vi "mtg reader - recolor file list.vi"(6 "max index":i32, 8 "rowsize":i32=6, 9 "Row":i32, 10 "Column":i32, 11 "table ref":refnum<vi>) -> (2 "slider pos":i32, 3 "table ref out":refnum<vi>)   [LabVIEW 2025]
uses:
  <vilib>/Utility/miscctls.llb/LVRowAndColumnTypeDef.ctl
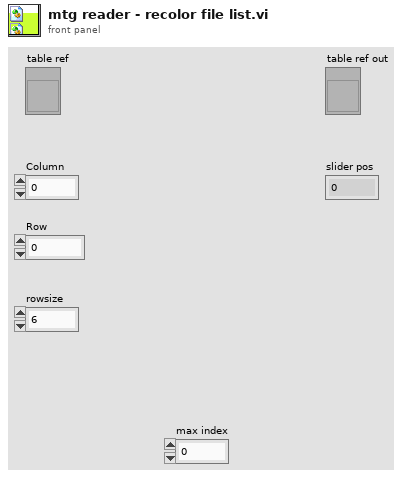
[diagram p1: front panel]
types:
  T1 = typedef "LVRowAndColumnTypeDef.ctl" = cluster{"Row":i32, "Column":i32}
  T2 = typedef "LVRowAndColumnUnsignedTypeDef.ctl" = cluster{"Row":u32, "Column":u32}
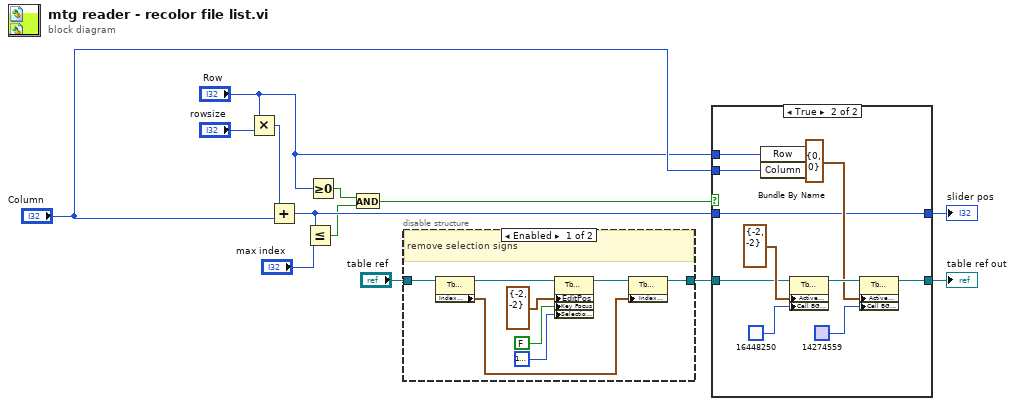
[diagram p0: block diagram]
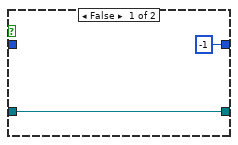
[diagram p3: hidden frame]
diagram:
  n1 = Multiply(x="Row", y="rowsize") -> (x*y=w12:i32)
  n2 = Add(x=w12, y="Column") -> (x+y=w9:i32)
  n3 = Less Or Equal?(x=w9, y="max index") -> (x <= y?=w5:bool)
  n4 = Greater Or Equal To 0?(x="Row") -> (x >= 0?=w4:bool)
  n5 = And(x=w4, y=w5) -> (x .and. y?=w6:bool)
  n6 = disable-structure shown="Enabled" {
    disable-tunnel: "table ref" -> [w18 w22]
    disable-tunnel: [w15 w22] -> w1
    frame Enabled {
      # "remove selection signs"
      n7 = property class="Tbl (strict)"(reference=w18) -> (reference out=w17:refnum<vi>, "Index Values"=w14:T2)  [unwired: 1 in, 1 out]
      n8 = property class="Tbl (strict)"(reference=w17, "EditPos"=T1 {"Row"=-2, "Column"=-2} ("Edit Position"), "Key Focus"=FALSE, "Selection Color"=u32 16777216) -> (reference out=w16:refnum<vi>)  [unwired: 1 in, 1 out]
      n9 = property class="Tbl (strict)"(reference=w16, "Index Values"=w14) -> (reference out=w15:refnum<vi>)  [unwired: 1 in, 1 out]
    }
    frame Disabled {
    }
  }
  n10 = case shown="True" w6 {
    tunnel: w1 -> [w24 w25]
    tunnel: [w24 w29] -> w3
    tunnel: "Row" -> [_ w28]
    tunnel: "Column" -> [_ w27]
    tunnel: w9 -> [_ w26]
    tunnel: [-1 w26] -> w8
    frame False {
    }
    frame True {
      n11 = Bundle By Name(cluster=T1 {"Row"=0, "Column"=0} ("Active Cell:Active Cell"), "Row"=w28, "Column"=w27) -> (w34:T1)
      n12 = property class="Tbl (strict)"(reference=w25, "Active Cell"=T1 {"Row"=-2, "Column"=-2} ("Active Cell:Active Cell"), "Cell BG Color"=u32 16448250 ("Active Cell:Cell Background Color")) -> (reference out=w35:refnum<vi>)  [unwired: 1 in, 1 out]
      n13 = property class="Tbl (strict)"(reference=w35, "Active Cell"=w34, "Cell BG Color"=u32 14274559 ("Active Cell:Cell Background Color")) -> (reference out=w29:refnum<vi>)  [unwired: 1 in, 1 out]
    }
  }
  "table ref out" <- w3
  "slider pos" <- w8
